vi "LabviewIngestService IngestDataStreamString Write.vi"(8 "error in":errorcluster, 10 "Request Data":T1, 11 "Call ID in":T3) -> (0 "error out":errorcluster, 2 "Success":bool, 3 "Call ID":T3)   [LabVIEW 2024, in "SiftProxy_client.lvlib"]
uses:
  SiftProxy_client.lvlib
  <vilib>/gRPC/LabVIEW gRPC Library/Shared/grpcId.ctl
  RPC Messages/sift_proxy_v1_IngestDataStreamStringRequest.ctl
  RPC Messages/google_protobuf_Timestamp.ctl
  9647bdd3-bda2-4565-bbb9-d670be58a455.vi
  RPC Messages/RichToFlatgoogle_protobuf_Timestamp.vi
  <vilib>/gRPC/LabVIEW gRPC Library/Shared/TranslateGrpcError.vi
  <vilib>/gRPC/LabVIEW gRPC Library/Server API/Server/Get Server DLL Path.vi
  <vilib>/Utility/error.llb/Error Cluster From Error Code.vi
  <vilib>/gRPC/LabVIEW gRPC Library/grpc-lvsupport-release.lvlib
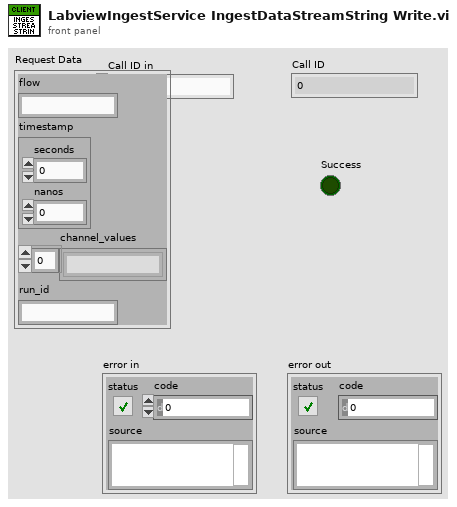
[diagram p1: front panel]
types:
  T1 = typedef "SiftProxy_client.lvlib/sift_proxy_v1_IngestDataStreamStringRequest.ctl" = cluster{"flow":string, "timestamp":T2, "channel_values":string[], "run_id":string}
  T2 = typedef "SiftProxy_client.lvlib/google_protobuf_Timestamp.ctl" = cluster{"seconds":i64, "nanos":i32}
  T3 = typedef "grpc-lvsupport-release.lvlib/grpcId.ctl" = u64
  T4 = typedef "SiftProxy_client.lvlib/sift_proxy_v1_IngestDataStreamStringRequest_Flat.ctl" = cluster{"flow":string, "timestamp":T5, "channel_values":string[], "run_id":string}
  T5 = typedef "SiftProxy_client.lvlib/google_protobuf_Timestamp_Flat.ctl" = cluster{"seconds":i64, "nanos":i32}
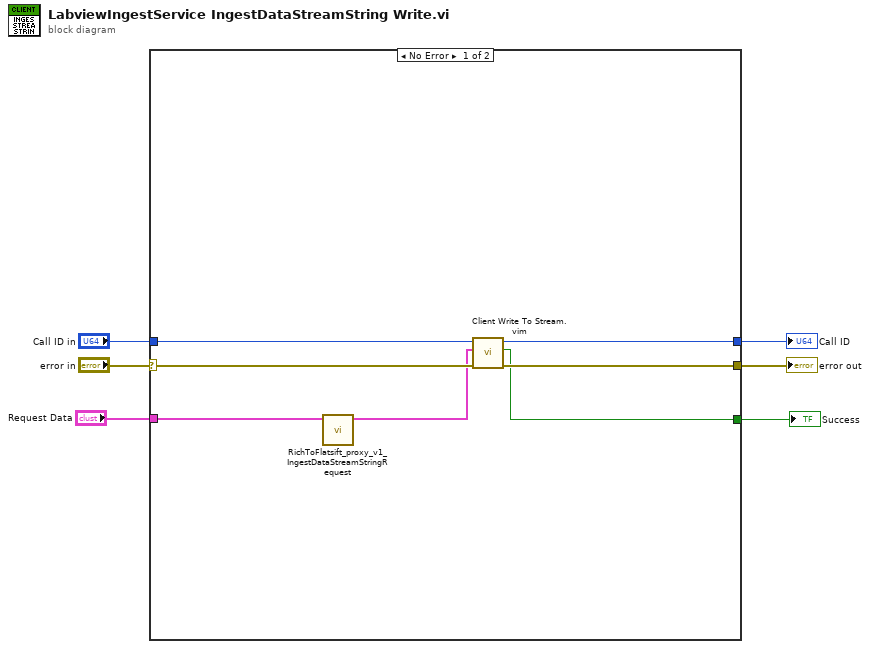
[diagram p0: block diagram]
diagram:
  n1 = case shown="No Error" "error in" {
    selector: "error in" -> [w13 w14]
    tunnel: [w12 w14] -> w5
    tunnel: "Call ID in" -> [w11 w15]
    tunnel: [w10 w15] -> w3
    tunnel: "Request Data" -> [w8 _]
    tunnel: [w9 _] -> w1
    frame No Error {
      n2 = call "RichToFlatsift_proxy_v1_IngestDataStreamStringRequest.vi"("InputCluster"=w8) -> ("OutputCluster"=w7:T4)  [unwired: 10 in]
      n3 = call "Client Write To Stream.vim"("error in"=w13, "Request Data"=w7, "Call ID in"=w11) -> ("error out"=w12:errorcluster, "Success"=w9:bool, "Call ID out"=w10:u64)  [unwired: 6 in]
    }
    frame Error {
    }
  }
  "error out" <- w5
  "Call ID" <- w3
  "Success" <- w1
